vi "Manually Update Data File.vi"() -> ()   [LabVIEW 2021]
uses:
  WPC Player and Financial Stats.ctl
panel:
  out "size(s)":i32[](array[numeric])
  out "Full WPC Stats":T1[][](array[typedef]) {"Date Updated" format="%<%m/%d/%Y>T"}
  in  "Update Stats Here":T1[][](array[typedef]) {"Date Updated" format="%<%m/%d/%Y>T"}
  out "error out":errorcluster
  in  "stop":bool
  in  "OK Button":bool
  in  "file path (use dialog)":path=path "C:/Users/manma/Google Drive/WPC Stat Scrape/Data/WPC Stats.bin"
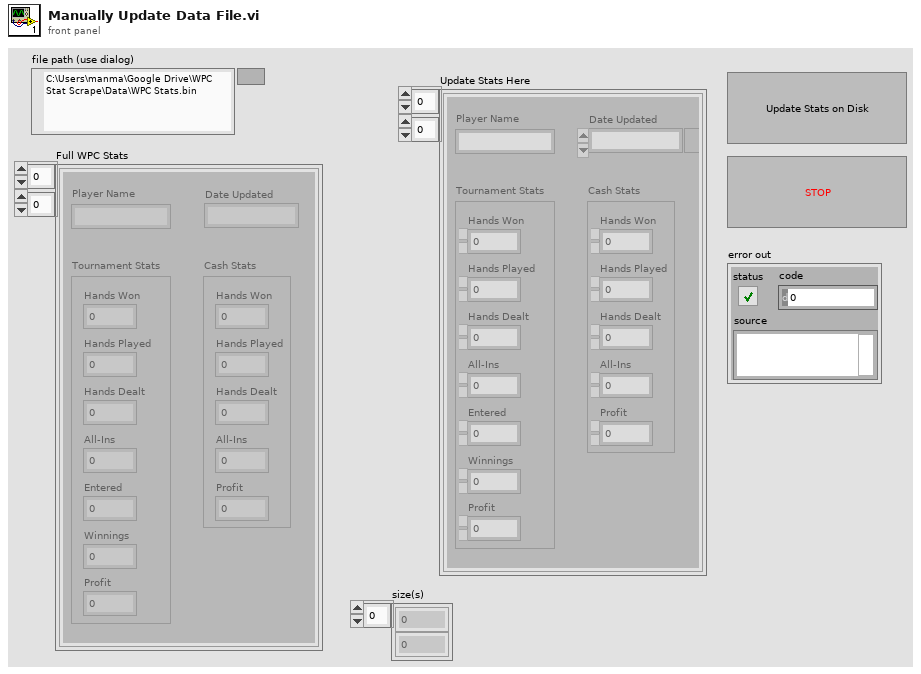
[diagram p1: front panel]
types:
  T1 = typedef "WPC Player and Financial Stats.ctl" = cluster{"Player Name":string, "Date Updated":timestamp, "Tournament Stats":cluster{"Hands Won":i32, "Hands Played":i32, "Hands Dealt":i32, "All-Ins":i32, "Entered":i32, "Winnings":dbl, "Profit":dbl}, "Cash Stats":cluster{"Hands Won":i32, "Hands Played":i32, "Hands Dealt":i32, "All-Ins":i32, "Profit":dbl}}
  T2 = enum16{"open", "replace", "create", "open or create", "replace or create", "replace or create with confirmation"}
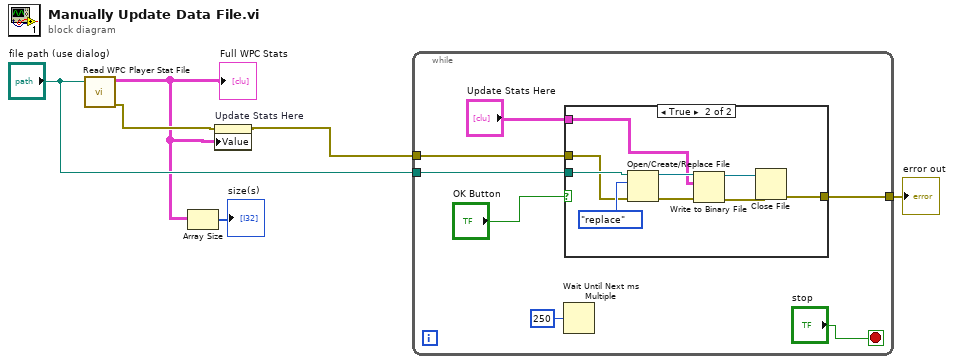
[diagram p0: block diagram]
diagram:
  n1 = call "Read WPC Player Stat File.vi"("file path (use dialog)"="file path (use dialog)") -> ("error out"=w4:errorcluster, "Full WPC Stats"=w2:T1[][])  [unwired: 8 in, 1 out]
  "Full WPC Stats" <- w2
  n2 = Array Size(array=w2) -> (size(s)=→"size(s)":i32[])
  n3 = property on="Update Stats Here" class="Arr (strict)"(error in=w4, "Value"=w2) -> (error out=w3:errorcluster)  [unwired: 1 in, 1 out]
  n4 = while {
    tunnel: "file path (use dialog)" -> [w10]
    tunnel: w3 -> [w9]
    tunnel: [w8] -> w5
    stop <- "stop" stop-if-true
    n5 = Wait Until Next ms Multiple(millisecond multiple=u32 250) -> ()  [unwired: 1 out]
    n6 = case shown="True" "OK Button" {
      tunnel: [_ w17] -> w8
      tunnel: w10 -> [_ w16]
      tunnel: "Update Stats Here" -> [_ w15]
      tunnel: w9 -> [_ w14]
      frame False {
      }
      frame True {
        n7 = Open/Create/Replace File(file path (use dialog)=w16, error in=w14, operation (0:open)=T2."replace") -> (refnum out=w20:refnum<file>, error out=w21:errorcluster)  [unwired: 3 in, 1 out]
        n8 = Write to Binary File(file (use dialog)=w20, data=w15, error in=w21) -> (refnum out=w19:refnum<file>, error out=w18:errorcluster)  [unwired: 3 in, 1 out]
        n9 = Close File(refnum=w19, error in=w18) -> (error out=w17:errorcluster)  [unwired: 1 out]
      }
    }
  }
  "error out" <- w5
